vi "Start Download.vi"(5 "Overall Status":refnum<vi>, 7 "Itemized Status":refnum<vi>, 8 "Error In":errorcluster, 11 "Dependecy Config":T2) -> (0 "Error Out":errorcluster, 2 "Install State":T1(ring), 3 "Dependecy Config":T2)   [LabVIEW 2011, in "LMH-Toolbox.lvlib" / "LMH-Installer Tools.lvlib"]
uses:
  LMH-Installer Tools.lvlib
  Type Defs/Dependency Config.ctl
  Type Defs/Dependecy.ctl
  Common/Private/Web/Type Defs/Download Task.ctl
  Common/LMH-Common.lvlib
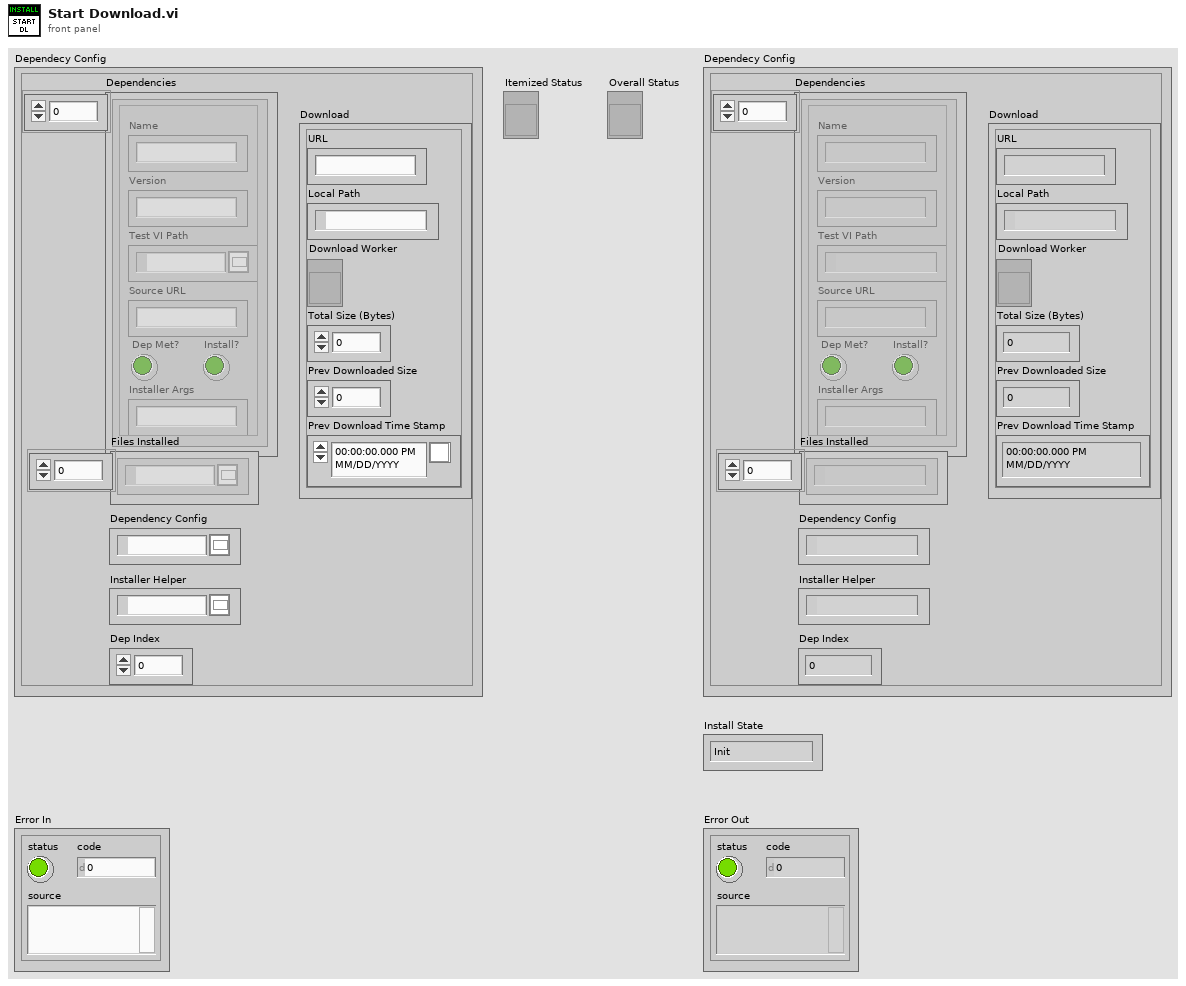
[diagram p1: front panel]
types:
  T1 = enum16{"Init", "Start DL", "Downloading", "DL Complete", "Done"}
  T2 = typedef "LMH-Toolbox.lvlib/LMH-Installer Tools.lvlib/Dependency Config.ctl" = cluster{"Dependencies":T3[], "Files Installed":path[], "Dependency Config":path, "Installer Helper":path, "Dep Index":i32, "Download":T4}
  T3 = typedef "LMH-Toolbox.lvlib/LMH-Installer Tools.lvlib/Dependecy.ctl" = cluster{"Name":string, "Version":string, "Test VI Path":path, "Source URL":string, "Dep Met?":bool, "Install?":bool, "Installer Args":string}
  T4 = typedef "LMH-Toolbox.lvlib/LMH-Common.lvlib/Download Task.ctl" = cluster{"URL":string, "Local Path":path, "Download Worker":refnum<vi>, "Total Size (Bytes)":u64, "Prev Downloaded Size":u64, "Prev Download Time Stamp":timestamp}
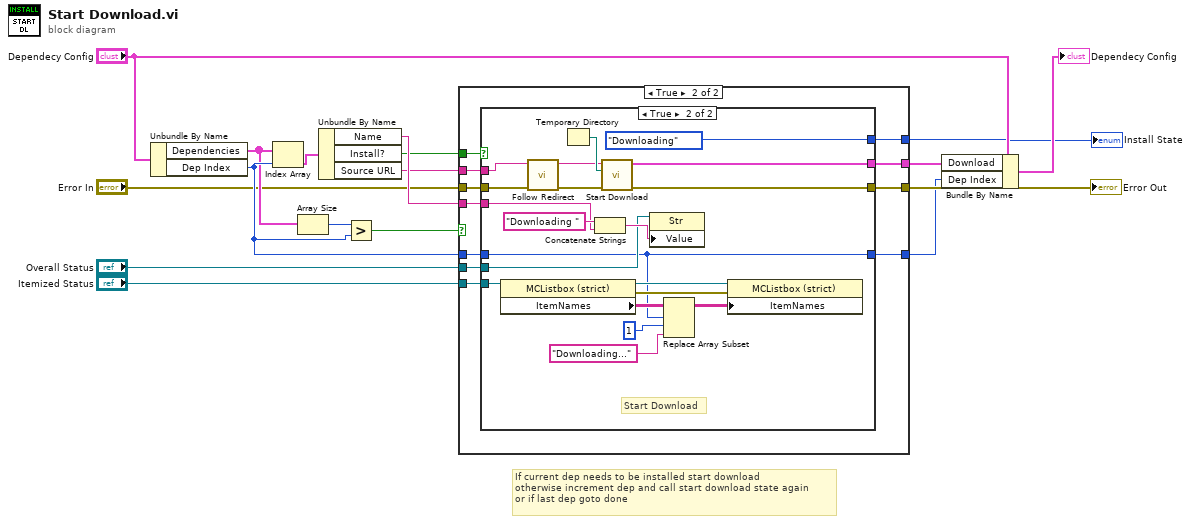
[diagram p0: block diagram]
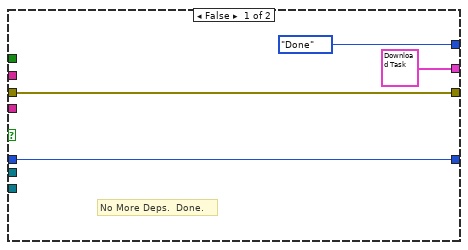
[diagram p2: hidden frame]
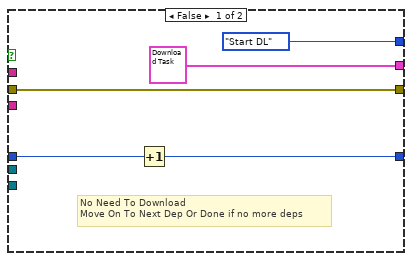
[diagram p3: hidden frame]
diagram:
  # "If current dep needs to be installed start download\notherwise increment dep and call start download state again \nor if last dep goto done"
  n1 = Unbundle By Name("Dependecy Config") -> ("Dependencies"=w13:T3[], "Dep Index"=w17:i32)
  n2 = Index Array(array=w13, index=w17) -> (element=w10:T3)
  n3 = Array Size(array=w13) -> (size(s)=w14:i32)
  n4 = Unbundle By Name(w10) -> ("Name"=w16:string, "Install?"=w11:bool, "Source URL"=w12:string)
  n5 = Greater?(x=w14, y=w17) -> (0:w15:bool)
  n6 = case shown="True" w15 {
    tunnel: "Error In" -> [w21 w32]
    tunnel: [w21 w31] -> w9
    tunnel: [T4 {"URL"="", "Local Path"=path "", "Download Worker"=refnum, "Total Size (Bytes)"=0, "Prev Downloaded Size"=0, "Prev Download Time Stamp"=timestamp(0 s since 1904-01-01)} ("Download") w30] -> w5
    tunnel: [T1."Done" ("Install State") w29] -> w2
    tunnel: w11 -> [_ w28]
    tunnel: w12 -> [_ w27]
    tunnel: w17 -> [w18 w26]
    tunnel: w16 -> [_ w25]
    tunnel: "Overall Status" -> [_ w24]
    tunnel: "Itemized Status" -> [_ w23]
    tunnel: [w18 w22] -> w1
    frame False {
      # "No More Deps.  Done."
    }
    frame True {
      n7 = case shown="True" w28 {
        tunnel: w27 -> [_ w38]
        tunnel: w32 -> [w37 w41]
        tunnel: [w37 w57] -> w31
        tunnel: [T4 {"URL"="", "Local Path"=path "", "Download Worker"=refnum, "Total Size (Bytes)"=0, "Prev Downloaded Size"=0, "Prev Download Time Stamp"=timestamp(0 s since 1904-01-01)} ("Download") w56] -> w30
        tunnel: w26 -> [w36 w42]
        tunnel: [T1."Start DL" ("Install State") T1."Downloading" ("Install State")] -> w29
        tunnel: w25 -> [_ w51]
        tunnel: w24 -> [_ w46]
        tunnel: w23 -> [_ w45]
        tunnel: [w33 w42] -> w22
        frame False {
          # "No Need To Download\nMove On To Next Dep Or Done if no more deps"
          n8 = Increment(x=w36) -> (x+1=w33:i32)
        }
        frame True {
          # "Start Download"
          n9 = property on="Property Node" class="MCListbox (strict)"(reference=w45) -> (reference out=w44:refnum<vi>, error out=w43:errorcluster, "ItemNames"=w50:string[][])  [unwired: 1 in]
          n10 = call "Follow Redirect.vi"("Error In"=w41, "URL"=w38) -> ("Error Out"=w40:errorcluster, "URL"=w39:string)  [unwired: 8 in]
          n11 = Temporary Directory() -> (w54:path)
          n12 = Concatenate Strings("Downloading " ("string"), w51) -> (w52:string)
          n13 = call "Start Download.vi"("Error In"=w40, "Download Directory"=w54, "URL"=w39) -> ("Error Out"=w57:errorcluster, "Download"=w56:T4)  [unwired: 7 in]
          n14 = property class="Str"(reference=w46, "Value"=w52) -> ()  [unwired: 1 in, 2 out]
          n15 = Replace Array Subset(array=w50, new element="Downloading..." ("new element/subarray"), index (row)=w42, index (col)=1 ("disabled index (row)")) -> (w49:string[][])
          n16 = property on="Property Node" class="MCListbox (strict)"(reference=w44, error in=w43, "ItemNames"=w49) -> ()  [unwired: 2 out]
        }
      }
    }
  }
  "Error Out" <- w9
  "Install State" <- w2
  n17 = Bundle By Name(cluster="Dependecy Config", "Download"=w5, "Dep Index"=w1) -> (→"Dependecy Config":T2)
